vi "CliConnectTo.vi"(0 "ref in":u64, 5 "Address":string, 7 "Rack":i32, 9 "Slot":i32, 11 "error in (no error)":errorcluster) -> (4 "ref out":u64, 6 "Result":i32, 15 "error out":errorcluster)   [LabVIEW 2020, in "Snap7.lvlib"]
uses:
  Snap7.lvlib
  windows/lv_snap7.dll
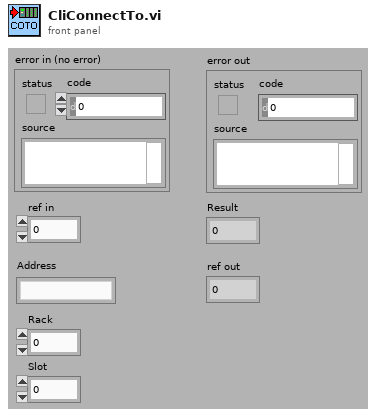
[diagram p1: front panel]
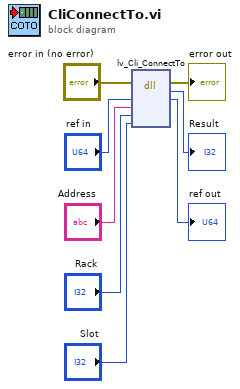
[diagram p0: block diagram]
diagram:
  n1 = dll-call lib="PTH2iabs CUsersFeng项目HLCEPS300-1老性能试验台SourcesSnap7libwindowslv_snap7.dll" fn="lv_Cli_ConnectTo"(error in="error in (no error)", "Client"="ref in", "Address"="Address", "Rack"="Rack", "Slot"="Slot") -> (error out=→"error out":errorcluster, "return type"=→"Result":i32, "Client"=→"ref out":u64)  [unwired: 5 in, 1 out]
